vi "test_click.vi"   [LabVIEW 2015]
uses:
  <vilib>/FieldPoint/Polymorphic Write.llb/FP Write (Float Array -IO).vi
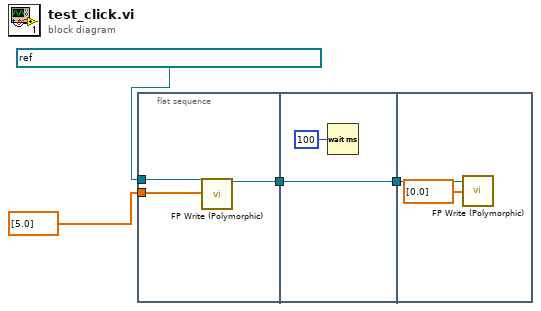
[diagram p0: block diagram]
diagram:
  n1 = flat-sequence {
    tunnel: refnum<k21> "sauna_fp\\FP @ 10_0_0_50\\cFP-AIO-610 @1\\Output 0" ("FieldPoint IO Point") -> [w5]
    tunnel: dbl[] [5.0] ("values") -> [w7]
    tunnel: [w6] -> w4
    tunnel: w4 -> [w8]
    tunnel: [w8] -> w3
    tunnel: w3 -> [w11]
    frame #0 {
      n2 = call-poly <vilib>:"FP Write (Polymorphic).vi"("FieldPoint IO Point In"=w5, "values"=w7) -> ("FieldPoint IO Point Out"=w6:refnum<k21>)  [unwired: 11 in, 2 out]
    }
    frame #1 {
      n3 = Wait (ms)(milliseconds to wait=u32 100) -> ()  [unwired: 1 out]
    }
    frame #2 {
      n4 = call-poly <vilib>:"FP Write (Polymorphic).vi"("FieldPoint IO Point In"=w11, "values"=dbl[] [0.0]) -> ()  [unwired: 11 in, 3 out]
    }
  }
